vi "SetPortGV.vi"(10 "COM":refnum<visa-resource-name>[](array[refnum]), 11 "USB":string[](array[string])) -> ()   [LabVIEW 2013]
uses:
  GlobalValue.vi
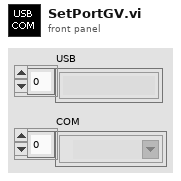
[diagram p1: front panel]
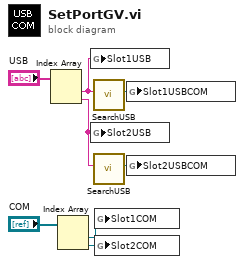
[diagram p0: block diagram]
diagram:
  n1 = Index Array(array="USB") -> (element #1=w6:string, element #2=w8:string)  [unwired: 2 in]
  n2 = Index Array(array="COM") -> (element #1=w2:refnum<visa-resource-name>, element #2=w3:refnum<visa-resource-name>)  [unwired: 2 in]
  n3 = global write "GlobalValue.vi" "Slot1USB"(w6) -> ()
  n4 = global write "GlobalValue.vi" "Slot2USB"(w8) -> ()
  n5 = call "SearchUSB.vi"("USB"=w6) -> ("USBPort"=w5:refnum<visa-resource-name>)  [unwired: 9 in, 1 out]
  n6 = call "SearchUSB.vi"("USB"=w8) -> ("USBPort"=w7:refnum<visa-resource-name>)  [unwired: 9 in, 1 out]
  n7 = global write "GlobalValue.vi" "Slot1COM"(w2) -> ()
  n8 = global write "GlobalValue.vi" "Slot2COM"(w3) -> ()
  n9 = global write "GlobalValue.vi" "Slot1USBCOM"(w5) -> ()
  n10 = global write "GlobalValue.vi" "Slot2USBCOM"(w7) -> ()
